vi "Disconnect.vi"(8 "error in":errorcluster, 11 "3300 in":refnum<class "3300.lvclass">) -> (0 "error out":errorcluster, 3 "3300 out":refnum<class "3300.lvclass">)   [LabVIEW 2019, in "3300.lvlib" / "3300.lvclass"]
uses:
  Library/3300.lvclass
  Library/3300.lvclass/3300.ctl
  builds/Instruments/Electronic Load.lvlibp/Library/Electronic Load.lvclass
  <instrlib>/Agilent N330X Series/Agilent N330X Series.lvlib
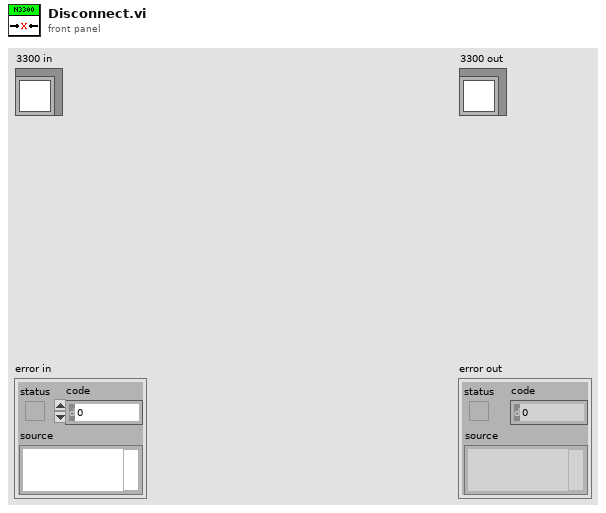
[diagram p1: front panel]
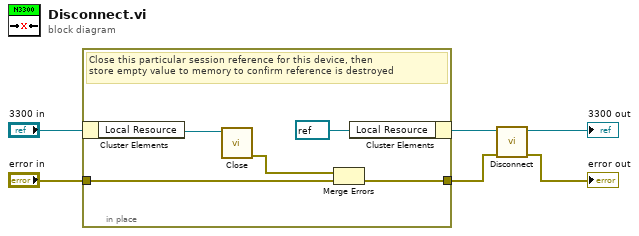
[diagram p0: block diagram]
diagram:
  n1 = in-place {
    in-place-border: "error in" -> [w10]
    in-place-border: [w8] -> w2
    # "Close this particular session reference for this device, then\nstore empty value to memory to confirm reference is destroyed"
    n2 = in-place-cluster #1("3300 in") -> ("Local Resource"=w11:refnum<visa-resource-name>)
    n3 = call <instrlib>:"Close.vi"("VISA resource name"=w11) -> ("error out"=w9:errorcluster)  [unwired: 10 in]
    n4 = Merge Errors(w9, w10) -> (w8:errorcluster)
    n5 = in-place-cluster #1("Local Resource"=refnum<visa-resource-name> refnum) -> (w4:refnum<class "3300.lvclass">)
  }
  n6 = call-parent "Disconnect.vi"("error in"=w2, "Electronic Load in"=w4) -> ("error out"=→"error out":errorcluster, "Electronic Load out"=→"3300 out":refnum<class "3300.lvclass">)  [unwired: 8 in]
